vi "Configure Waveform.vi"(8 "error in (no error)":errorcluster, 10 "Params":variant, 11 "NI DMM in":refnum<class "NI DMM.lvclass">) -> (0 "error out":errorcluster, 3 "NI DMM out":refnum<class "NI DMM.lvclass">)   [LabVIEW 2020, in "NI DMM.lvlib" / "NI DMM.lvclass"]
uses:
  NI DMM.lvclass
  NI DMM.lvclass/NI DMM.ctl
  TypeDefs/DMM waveform settings.ctl
  <instrlib>/niDMM/nidmm.llb/niDMM Waveform Function.ctl
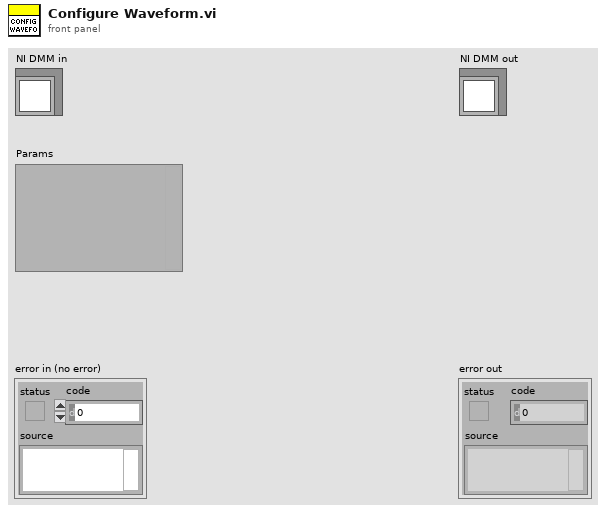
[diagram p1: front panel]
types:
  T1 = typedef "NI DMM.lvlib/NI DMM.lvclass/DMM waveform settings.ctl" = cluster{"Waveform Points":i32, "Function":T2, "Rate":dbl, "Range":dbl, "Settle Time":dbl}
  T2 = typedef "niDMM Waveform Function.ctl" = i32
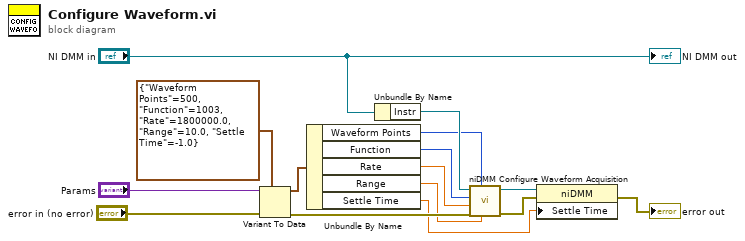
[diagram p0: block diagram]
diagram:
  n1 = Variant To Data(error in="error in (no error)", type=T1 {"Waveform Points"=500, "Function"=1003, "Rate"=1800000.0, "Range"=10.0, "Settle Time"=-1.0}, Variant="Params") -> (data=w6:T1, error out=w9:errorcluster)
  n2 = Unbundle By Name(w6) -> ("Waveform Points"=w3:i32, "Function"=w2:T2, "Rate"=w4:dbl, "Range"=w5:dbl, "Settle Time"=w1:dbl)
  n3 = Unbundle By Name("NI DMM in") -> ("Instr"=w13:refnum<k15>)
  n4 = call <instrlib>:"niDMM Configure Waveform Acquisition.vi"("Range"=w5, "Waveform Points"=w3, "error in (no error)"=w9, "Rate"=w4, "Function"=w2, "instrument handle"=w13) -> ("error out"=w12:errorcluster, "instrument handle out"=w15:refnum<k15>)  [unwired: 4 in]
  n5 = property class="niDMM"(reference=w15, error in=w12, "Settle Time"=w1) -> (error out=→"error out":errorcluster)  [unwired: 1 out]
  "NI DMM out" <- "NI DMM in"
